vi "Sim Data.vi"() -> ()   [LabVIEW 2024]
panel:
  in  "x .or. y?":bool
  out "Received Data 2":dbl(graph)
  out "Received Data":dbl(graph)
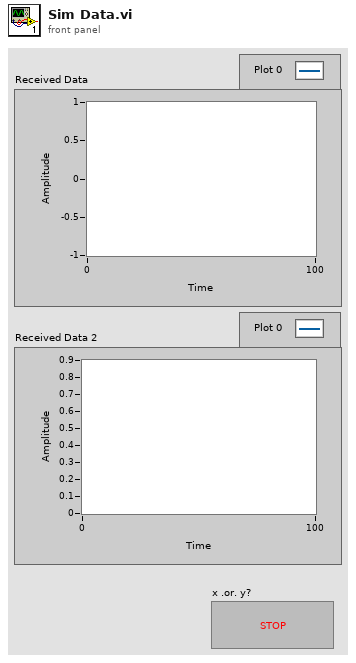
[diagram p1: front panel]
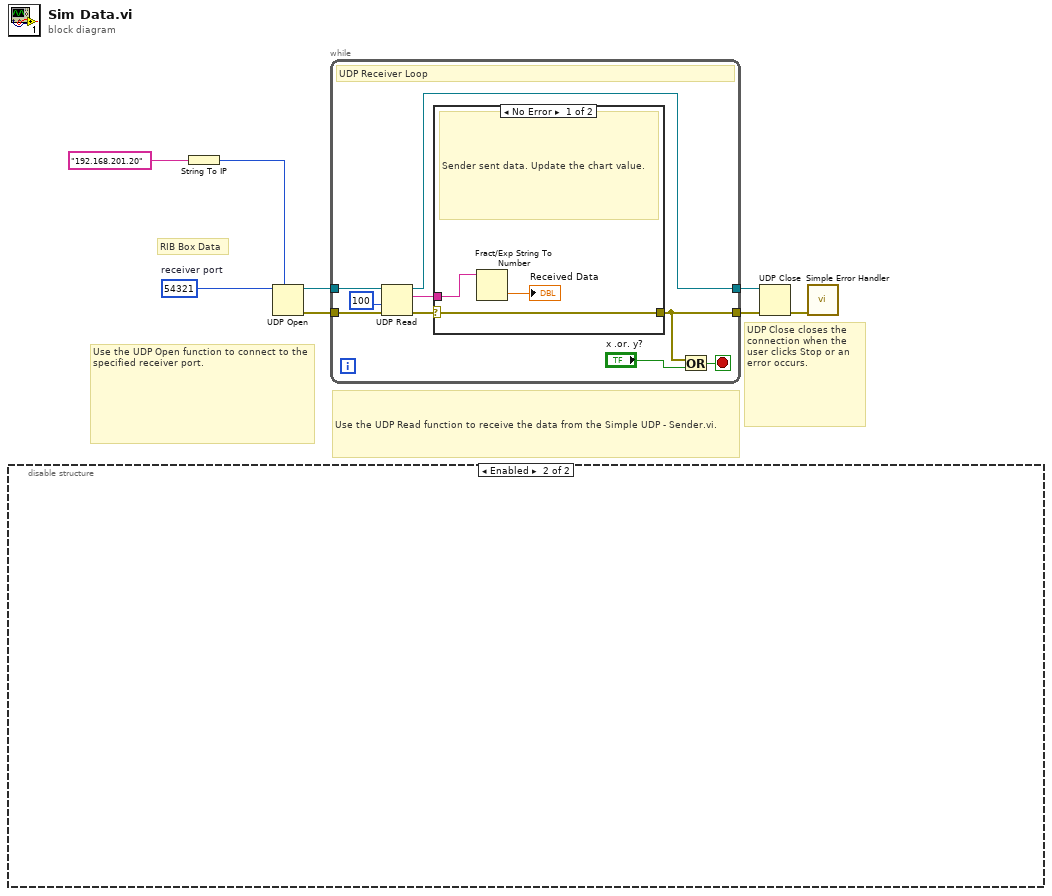
[diagram p0: block diagram]
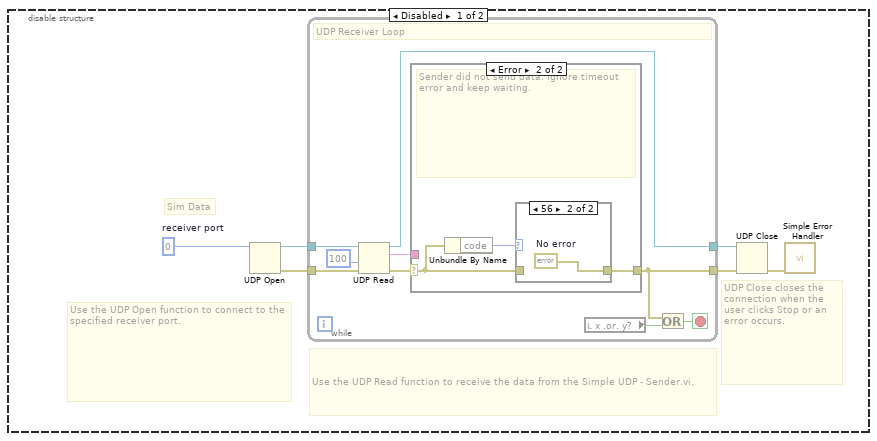
[diagram p2: hidden frame]
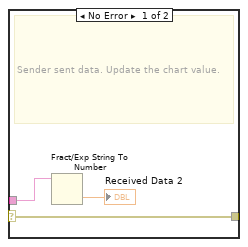
[diagram p3: hidden frame]
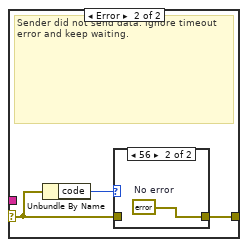
[diagram p5: hidden frame]
diagram:
  w3 = u16 54321  # receiver port
  # "RIB Box Data"
  # "UDP Close closes the connection when the user clicks Stop or an error occurs."
  # "Use the UDP Open function to connect to the specified receiver port."
  # "Use the UDP Read function to receive the data from the Simple UDP - Sender.vi."
  n1 = disable-structure shown="Enabled" {
    frame Disabled {
      w9 = u16 0  # receiver port
      # "Sim Data"
      # "UDP Close closes the connection when the user clicks Stop or an error occurs."
      # "Use the UDP Open function to connect to the specified receiver port."
      # "Use the UDP Read function to receive the data from the Simple UDP - Sender.vi."
      n2 = UDP Open(11:w9) -> (port=w10:refnum<k16>, 0:w11:errorcluster)  [unwired: 4 in, 1 out]
      n3 = while {
        tunnel: w10 -> [w23]
        tunnel: [w16] -> w14
        tunnel: w11 -> [w21]
        tunnel: [w17] -> w12
        stop <- w22 stop-if-true
        # "UDP Receiver Loop"
        n4 = UDP Read(connection ID=w23, timeout ms (25000)=100, 8:w21) -> (data out=w19:string, error out=w18:errorcluster, 3:w16:refnum<k16>)  [unwired: 3 out]
        n5 = case shown="Error" w18 {
          selector: w18 -> [w24 w28]
          tunnel: w19 -> [w26 _]
          tunnel: [w24 w27] -> w17
          frame No Error {
            # "Sender sent data. Update the chart value."
            n6 = Fract/Exp String To Number(string=w26) -> (number=→"Received Data 2":dbl)  [unwired: 3 in, 1 out]
          }
          frame Error {
            # "Sender did not send data. Ignore timeout error and keep waiting."
            n7 = Unbundle By Name(w28) -> ("code"=w29:i32)
            n8 = case shown="56" w29 {
              tunnel: w28 -> [w30 _]
              tunnel: [w30 w31] -> w27
              frame Default {
              }
              frame 56 {
                w31 = errorcluster {"status"=FALSE, "code"=0, "source"=""}  # No error
              }
            }
          }
        }
        n9 = local read "x .or. y?"() -> (w15:bool)
        n10 = Or(x=w17, y=w15) -> (x .or. y?=w22:bool)
      }
      n11 = UDP Close(connection ID=w14, 8:w12) -> (error out=w13:errorcluster)  [unwired: 1 out]
      n12 = call <vilib>:"Simple Error Handler.vi"("error in (no error)"=w13) -> ()  [unwired: 1 in, 8 out]
    }
    frame Enabled {
    }
  }
  n13 = String To IP(1:"192.168.201.20" ("name")) -> (0:w1:u32)
  n14 = UDP Open(7:w1, 11:w3) -> (port=w4:refnum<k16>, 0:w5:errorcluster)  [unwired: 3 in, 1 out]
  n15 = while {
    tunnel: w4 -> [w40]
    tunnel: [w34] -> w8
    tunnel: w5 -> [w39]
    tunnel: [w35] -> w6
    stop <- w33 stop-if-true
    # "UDP Receiver Loop"
    n16 = UDP Read(connection ID=w40, timeout ms (25000)=100, 8:w39) -> (data out=w37:string, error out=w36:errorcluster, 3:w34:refnum<k16>)  [unwired: 3 out]
    n17 = case shown="No Error" w36 {
      selector: w36 -> [w41 w45]
      tunnel: w37 -> [w43 _]
      tunnel: [w41 w44] -> w35
      frame No Error {
        # "Sender sent data. Update the chart value."
        n18 = Fract/Exp String To Number(string=w43) -> (number=→"Received Data":dbl)  [unwired: 3 in, 1 out]
      }
      frame Error {
        # "Sender did not send data. Ignore timeout error and keep waiting."
        n19 = Unbundle By Name(w45) -> ("code"=w46:i32)
        n20 = case shown="56" w46 {
          tunnel: w45 -> [w47 _]
          tunnel: [w47 w48] -> w44
          frame Default {
          }
          frame 56 {
            w48 = errorcluster {"status"=FALSE, "code"=0, "source"=""}  # No error
          }
        }
      }
    }
    n21 = Or(x=w35, y="x .or. y?") -> (x .or. y?=w33:bool)
  }
  n22 = UDP Close(connection ID=w8, 8:w6) -> (error out=w7:errorcluster)  [unwired: 1 out]
  n23 = call <vilib>:"Simple Error Handler.vi"("error in (no error)"=w7) -> ()  [unwired: 1 in, 8 out]
